vi "THzTimeAutoSave.vi"(0 "Numeric":i32, 1 "x-axis":sgl[](array[numeric]), 2 "y-axis":dbl[](array[numeric]), 3 "Autosave Directory for Long-term Average Scan":path) -> ()   [LabVIEW 2010]
uses:
  <vilib>/Utility/file.llb/Write To Spreadsheet File (DBL).vi
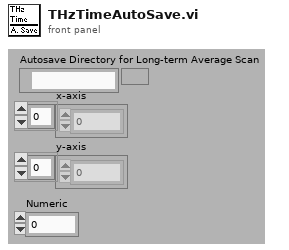
[diagram p1: front panel]
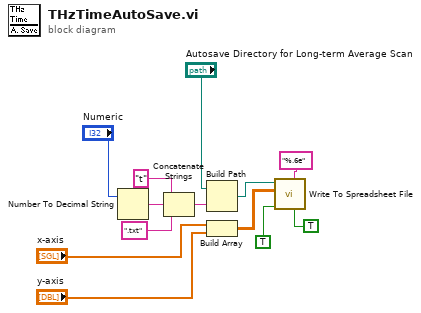
[diagram p0: block diagram]
diagram:
  n1 = Number To Decimal String(number="Numeric") -> (decimal integer string=w3:string)  [unwired: 1 in]
  n2 = Concatenate Strings("t" ("string"), w3, ".txt" ("string")) -> (w7:string)
  n3 = Build Path(base path="Autosave Directory for Long-term Average Scan", name or relative path=w7) -> (appended path=w13:path)
  n4 = Build Array("x-axis", "y-axis") -> (w12:dbl[][])
  n5 = call-poly <vilib>:"Write To Spreadsheet File.vi"("transpose? (no:F)"=TRUE ("transpose?\n(no:F)"), "format (%.3f)"="%.6e", "append to file? (new file:F)"=TRUE ("transpose?\n(no:F)"), "2D data"=w12, "file path (dialog if empty)"=w13) -> ()  [unwired: 3 in, 1 out]
